vi "SwerveKinematics_ToSwerveModuleStates.vi"(9 "CenterOfRotation":T3={"X"=0.0, "Y"=1.0} {"Y" format="%14.3f"; "X" format="%14.3f"}, 10 "ChassisSpeeds":T6 {"vOmega" format="%10.3f"; "vY" format="%10.3f"; "vX" format="%10.3f"}, 11 "in SWERVE_DRIVE_KINEMATICS":T4 {"PrevCoR"."Y" format="%14.3f"; "PrevCoR"."X" format="%14.3f"; "Modules"."Y" format="%14.3f"; "Modules"."X" format="%14.3f"}) -> (1 "ModuleStates":T1[](array[typedef]) {"Angle"."SIN" format="%13.4f"; "Angle"."COS" format="%13.4f"; "Angle"."VALUE" format="%13.4f"}, 3 "out SWERVE_DRIVE_KINEMATICS":T4 {"PrevCoR"."Y" format="%14.3f"; "PrevCoR"."X" format="%14.3f"; "Modules"."Y" format="%14.3f"; "Modules"."X" format="%14.3f"})   [LabVIEW 2019, in "Trajectory_Library.lvlib"]
doc: "Performs inverse kinematics to return the module states from a desired chassis velocity. This method is often used to convert joystick values into module speeds and angles.\n \nThis function also supports variable centers of rotation. During normal operations, the center of rotation is usually the same as the physical center of the robot; therefore, the argument is defaulted to that use case. However, if you wish to change the center of rotation for evasive manuevers, vision alignment, or for any other use case, you can do so.\n \nParameters:\n - chassisSpeeds -- The desired chassis speed.\n - centerOfRotation -- The center of rotation. For example, if you set the center of rotation at one corner of the robot and provide a chassis speed that only has a dtheta component, the robot will rotate around that corner. (Meters)\n\nReturns:\n - ModuleStates - An array of data structures containing the module states. Use caution because these module states are not normalized. Sometimes, a user input may cause one of the module speeds to go above the attainable max velocity. Use the {@link #normalizeWheelSpeeds(SwerveModuleState[], double) normalizeWheelSpeeds} function to rectify this issue."
uses:
  Trajectory_Library.lvlib
  TypeDef/SWERVE_DRIVE_KINEMATICS.ctl
  <vilib>/Analysis/Matrix/Datatypes/RealMatrix.ctl
  TypeDef/TRANSLATION2D.ctl
  TypeDef/CHASSIS_SPEEDS.ctl
  TypeDef/SWERVE_DRIVE_MODULE_STATE.ctl
  TypeDef/ROTATION2D.ctl
  MatBuilder_Create.vi
  MatrixHelper_CoerceSize.vi
  <vilib>/Analysis/Matrix/Numeric/Multiply/Multiply - RM,RM.vi
  <vilib>/Analysis/Matrix/NI_Matrix.lvlib
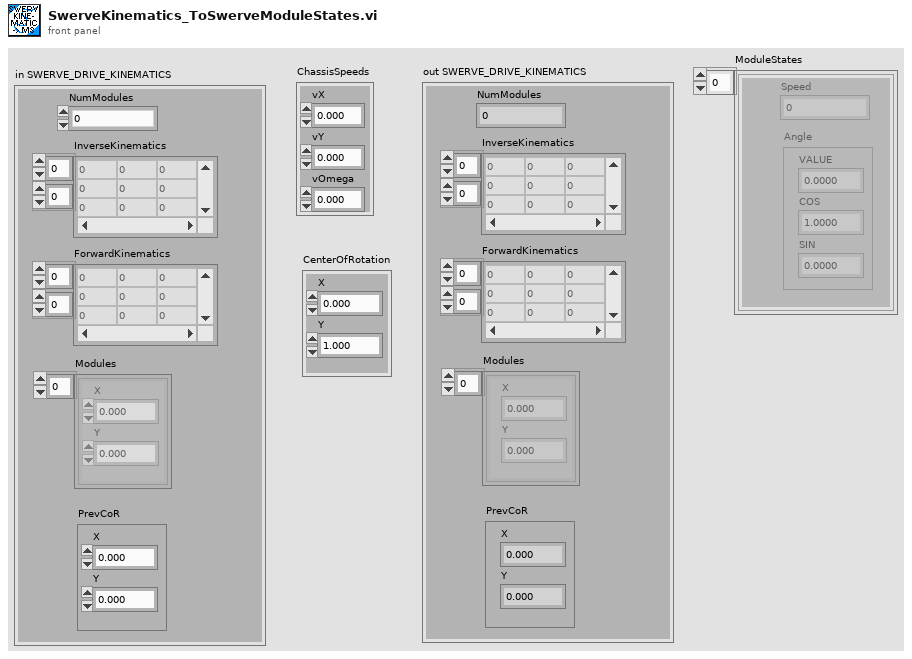
[diagram p1: front panel]
types:
  T1 = typedef "Trajectory_Library.lvlib/SWERVE_DRIVE_MODULE_STATE.ctl" = cluster{"Speed":dbl, "Angle":T2}
  T2 = typedef "Trajectory_Library.lvlib/ROTATION2D.ctl" = cluster{"VALUE":dbl, "COS":dbl, "SIN":dbl}
  T3 = typedef "Trajectory_Library.lvlib/TRANSLATION2D.ctl" = cluster{"X":dbl, "Y":dbl}
  T4 = typedef "Trajectory_Library.lvlib/SWERVE_DRIVE_KINEMATICS.ctl" = cluster{"NumModules":i32, "InverseKinematics":T5, "ForwardKinematics":T5, "Modules":T3[], "PrevCoR":T3}
  T5 = typedef "NI_Matrix.lvlib/RealMatrix.ctl" = dbl[][]
  T6 = typedef "Trajectory_Library.lvlib/CHASSIS_SPEEDS.ctl" = cluster{"vX":dbl, "vY":dbl, "vOmega":dbl}
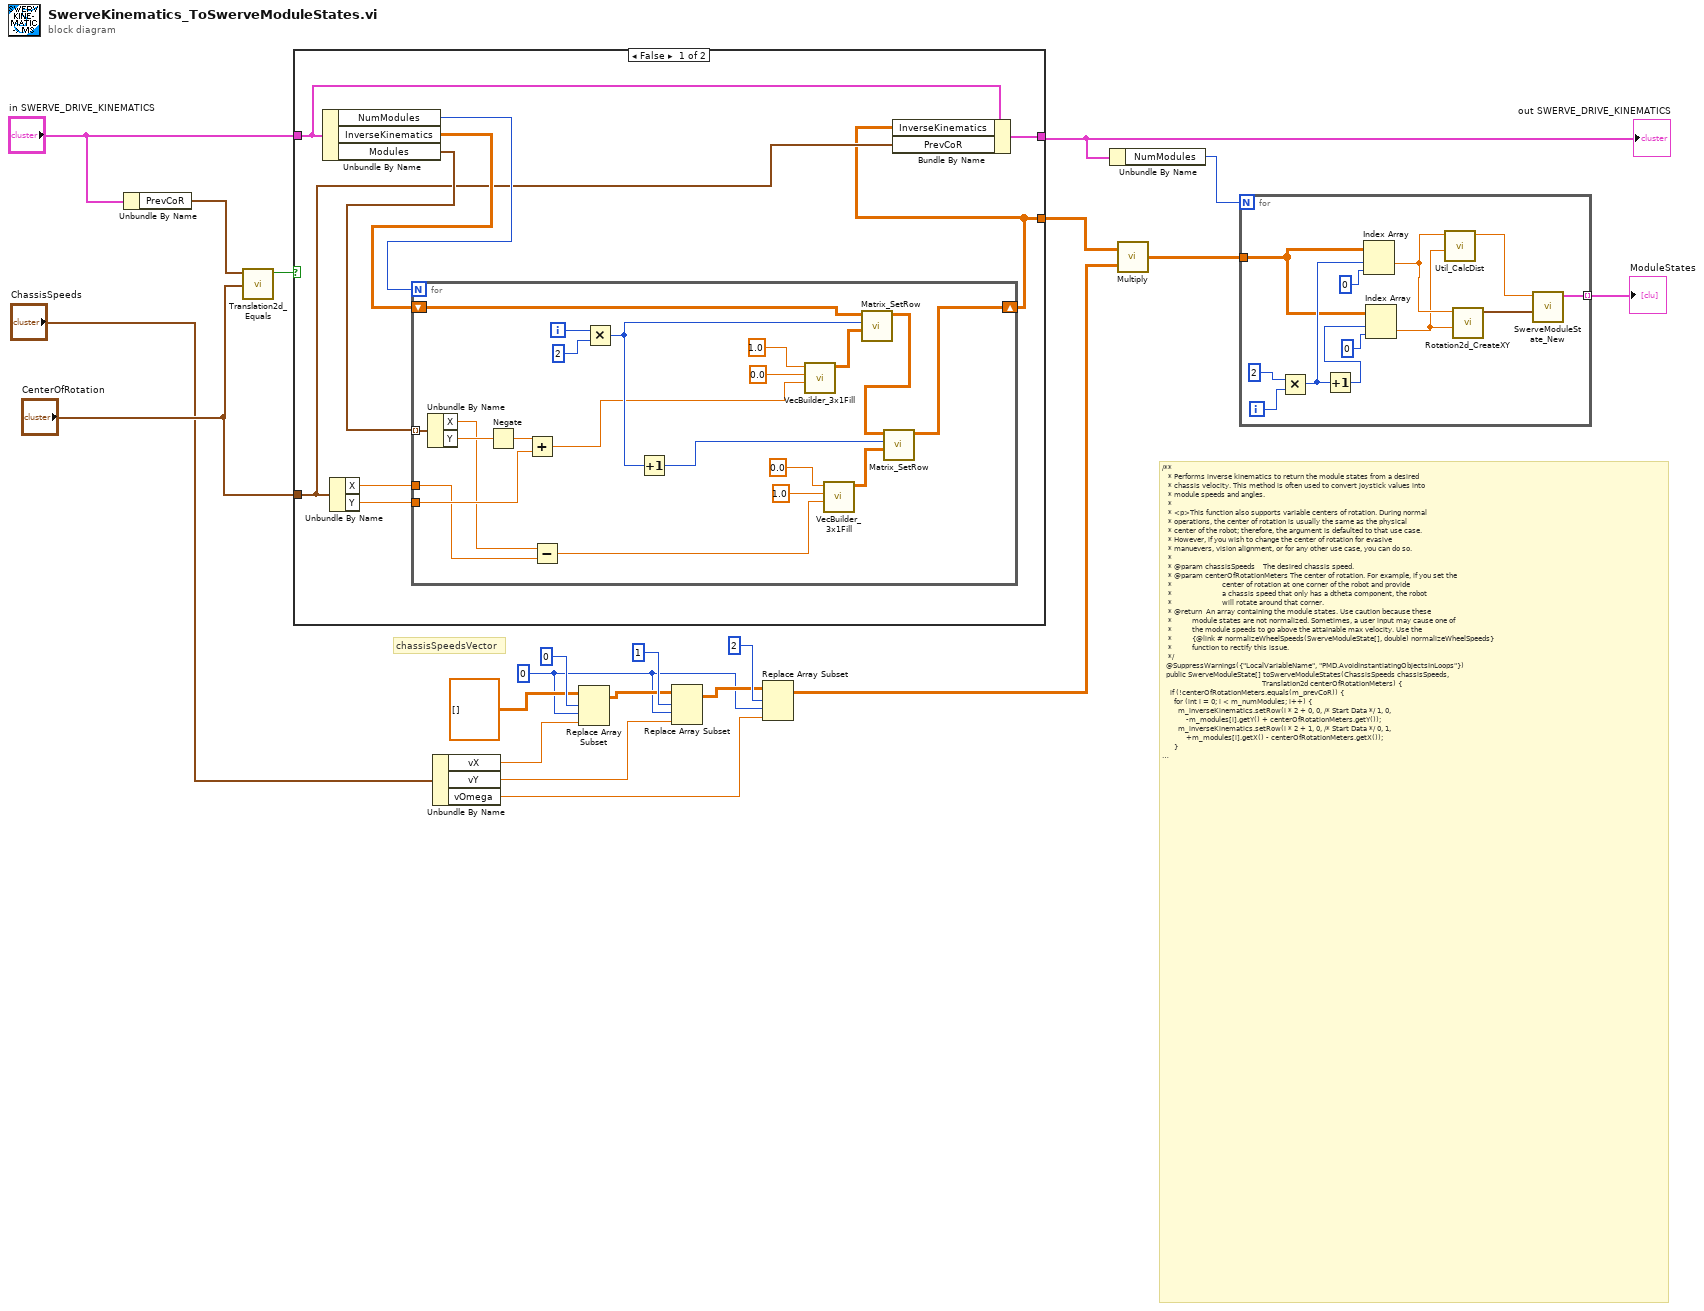
[diagram p0: block diagram]
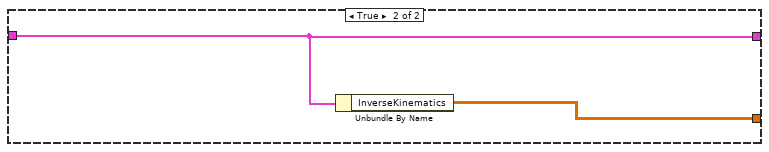
[diagram p2: hidden frame]
diagram:
  w11 = 0 ("disabled index (col)")
  # "chassisSpeedsVector"
  # "/**\n   * Performs inverse kinematics to return the module states from a desired\n   * chassis velocity. This method is often used to convert joystick values into\n   * module speeds and angles.\n   *\n   * <p>This function also supports variable centers of rotation. During normal\n   * operations, the center of rotation is usually the same as the physical\n   * center of the robot; therefore, the argument is defaulted to that use case.\n   * However, if you wish to change the center of rotation for evasive\n   * manuevers, vision alignment, or for any other use case, you can do so.\n   *\n   * @param chassisSpeeds    The desired chassis speed.\n   * @param centerOfRotationMeters The center of rotation. For example, if you set the\n   *                         center of rotation at one corner of the robot and provide\n   *                         a chassis speed that only has a dtheta component, the robot\n   *                         will rotate around that corner.\n   * @return  An array containing the module states. Use caution because these\n   *          module states are not normalized. Sometimes, a user input may cause one of\n   *          the module speeds to go above the attainable max velocity. Use the\n   *          {@link # normalizeWheelSpeeds(SwerveModuleState[], double) normalizeWheelSpeeds}\n   *          function to rectify this issue.\n   */\n  @SuppressWarnings({\"LocalVariableName\", \"PMD.AvoidInstantiatingObjectsInLoops\"})\n  public SwerveModuleState[] toSwerveModuleStates(ChassisSpeeds chassisSpeeds,\n                                                  Translation2d centerOfRotationMeters) {\n    if (!centerOfRotationMeters.equals(m_prevCoR)) {\n      for (int i = 0; i < m_numModules; i++) {\n        m_inverseKinematics.setRow(i * 2 + 0, 0, /* Start Data */ 1, 0,\n            -m_modules[i].getY() + centerOfRotationMeters.getY());\n        m_inverseKinematics.setRow(i * 2 + 1, 0, /* Start Data */ 0, 1,\n            +m_modules[i].getX() - centerOfRotationMeters.getX());\n      }\n      m_prevCoR = centerOfRotationMeters;\n    }\n\n    var chassisSpeedsVector = new SimpleMatrix(3, 1);\n    chassisSpeedsVector.setColumn(0, 0,\n        chassisSpeeds.vxMetersPerSecond, chassisSpeeds.vyMetersPerSecond,\n        chassisSpeeds.omegaRadiansPerSecond);\n\n    var moduleStatesMatrix = m_inverseKinematics.mult(chassisSpeedsVector);\n    SwerveModuleState[] moduleStates = new SwerveModuleState[m_numModules];\n\n    for (int i = 0; i < m_numModules; i++) {\n      double x = moduleStatesMatrix.get(i * 2, 0);\n      double y = moduleStatesMatrix.get(i * 2 + 1, 0);\n\n      double speed = Math.hypot(x, y);\n      Rotation2d angle = new Rotation2d(x, y);\n\n      moduleStates[i] = new SwerveModuleState(speed, angle);\n    }\n\n    return moduleStates;\n  }"
  n1 = Unbundle By Name("in SWERVE_DRIVE_KINEMATICS") -> ("PrevCoR"=w21:T3)
  n2 = call "Translation2d_Equals.vi"("other Translation"="CenterOfRotation", "In Translation"=w21) -> ("Equals"=w20:bool)  [unwired: 9 in]
  n3 = case shown="False" w20 {
    tunnel: "in SWERVE_DRIVE_KINEMATICS" -> [w24 w53]
    tunnel: [w25 w53] -> w4
    tunnel: "CenterOfRotation" -> [w23 _]
    tunnel: [w22 w52] -> w6
    frame False {
      n4 = Unbundle By Name(w24) -> ("NumModules"=w30:i32, "InverseKinematics"=w29:T5, "Modules"=w28:T3[])
      n5 = Unbundle By Name(w23) -> ("X"=w26:dbl, "Y"=w27:dbl)
      n6 = for {
        N: w30 -> [_]
        shift-right: [w31] -> w22
        shift-left: w29 -> [w32]
        tunnel: w28 -> [w49] mode=indexing
        tunnel: w27 -> [w46]
        tunnel: w26 -> [w44]
        i -> [w51]
        n7 = Unbundle By Name(w49) -> ("X"=w45:dbl, "Y"=w48:dbl)
        n8 = Negate(x=w48) -> (-x=w47:dbl)
        n9 = Add(x=w47, y=w46) -> (x+y=w34:dbl)
        n10 = Subtract(x=w45, y=w44) -> (x-y=w33:dbl)
        n11 = Multiply(x=w51, y=2) -> (x*y=w35:i32)
        n12 = Increment(x=w35) -> (x+1=w43:i32)
        n13 = call "VecBuilder_3x1Fill.vi"("R2"=w34, "R1"=0.0, "R0"=1.0) -> ("output matrix"=w41:T5)  [unwired: 8 in]
        n14 = call "VecBuilder_3x1Fill.vi"("R2"=w33, "R1"=1.0, "R0"=0.0) -> ("output matrix"=w40:T5)  [unwired: 8 in]
        n15 = call "Matrix_SetRow.vi"("Fill Row Vector"=w41, "Row"=w35, "input matrix"=w32) -> ("output matrix"=w42:T5)  [unwired: 7 in, 1 out]
        n16 = call "Matrix_SetRow.vi"("Fill Row Vector"=w40, "Row"=w43, "input matrix"=w42) -> ("output matrix"=w31:T5)  [unwired: 7 in, 1 out]
      }
      n17 = Bundle By Name(cluster=w24, "InverseKinematics"=w22, "PrevCoR"=w23) -> (w25:T4)
    }
    frame True {
      n18 = Unbundle By Name(w53) -> ("InverseKinematics"=w52:T5)
    }
  }
  "out SWERVE_DRIVE_KINEMATICS" <- w4
  n19 = Unbundle By Name("ChassisSpeeds") -> ("vX"=w9:dbl, "vY"=w8:dbl, "vOmega"=w7:dbl)
  n20 = Replace Array Subset(array=T5 [] ("InverseKinematics"), new element=w9, index (row)=0 ("disabled index (row)"), index (col)=w11) -> (w13:T5)
  n21 = Replace Array Subset(array=w13, new element=w8, index (row)=1 ("disabled index (row)"), index (col)=w11) -> (w12:T5)
  n22 = Replace Array Subset(array=w12, new element=w7, index (row)=2 ("disabled index (row)"), index (col)=w11) -> (w5:T5)
  n23 = Unbundle By Name(w4) -> ("NumModules"=w3:i32)
  n24 = call-poly <vilib>:"Multiply.vi"("Real Matrix B"=w5, "Real Matrix A"=w6) -> ("A * B"=w1:T5)
  n25 = for {
    N: w3 -> [_]
    tunnel: [w65] -> w2 mode=indexing
    tunnel: w1 -> [w58]
    i -> [w64]
    n26 = Multiply(x=2, y=w64) -> (x*y=w61:i32)
    n27 = Increment(x=w61) -> (x+1=w59:i32)
    n28 = Index Array(array=w58, index (row)=w61, index (col)=0) -> (element=w57:dbl)
    n29 = Index Array(array=w58, index (row)=w59, index (col)=0) -> (element=w56:dbl)
    n30 = call "Util_CalcDist.vi"("Y"=w56, "X"=w57) -> ("DIST"=w54:dbl)  [unwired: 9 in]
    n31 = call "Rotation2d_CreateXY.vi"("Y or sine"=w56, "X or  cosine"=w57) -> ("ROTATION"=w55:T2)  [unwired: 9 in]
    n32 = call "SwerveModuleState_New.vi"("ROTATION"=w55, "Speed"=w54) -> ("SWERVE_DRIVE_MODULE_STATE"=w65:T1)  [unwired: 9 in]
  }
  "ModuleStates" <- w2
